vi "Redetection_initial detectoin.vi"(6 "Sweep #":i32, 7 "File Paramters":T2, 9 "New Smoothing Parameter":T3, 10 "Data (1 sweep)":dbl[](array[numeric]), 11 "Polarity":T1 items=["Inward", "Outward"]) -> (1 "Sweep trace":cluster{dbl[], "X":dbl[]}[](array[cluster]), 2 "Detected event":cluster{dbl[][]}, 3 "Original trace (unfiltered)":cluster{dbl[], "Data (1 sweep) ":dbl[]})   [LabVIEW 2017]
uses:
  Polarity.ctl
  <vilib>/Analysis/3filter.llb/Savitzky-Golay Filter (DBL).vi
  <vilib>/addons/Wavelet Analysis/application.llb/WA Multiscale Peak Detection (Array).vi
  <vilib>/Analysis/NI_AALBase.lvlib
  <vilib>/addons/_Advanced Signal Processing/NI_AdvSigProcWA.lvlib
  <vilib>/Analysis/NI_AALPro.lvlib
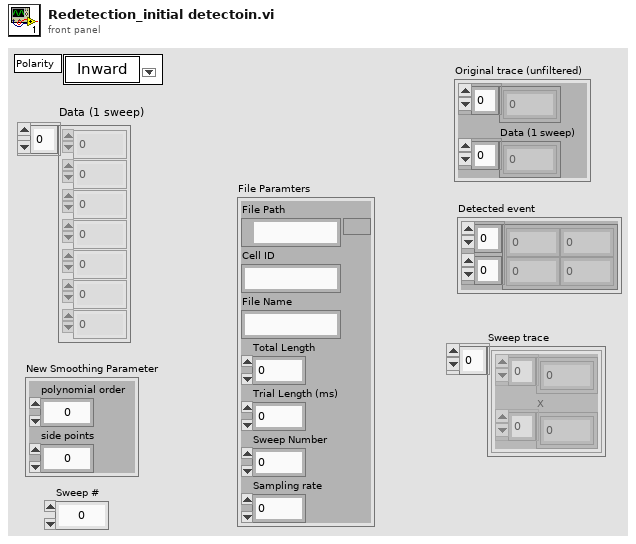
[diagram p1: front panel]
types:
  T1 = typedef "Polarity.ctl" = u16
  T2 = cluster{"File Path":path, "Cell ID":string, "File Name":string, "Total Length":i32, "Trial Length (ms)":dbl, "Sweep Number":dbl, "Sampling rate":dbl}
  T3 = cluster{"polynomial order":i32, "side points":i32}
  T4 = cluster{"detrend? (F)":bool, "threshold frequency":dbl}
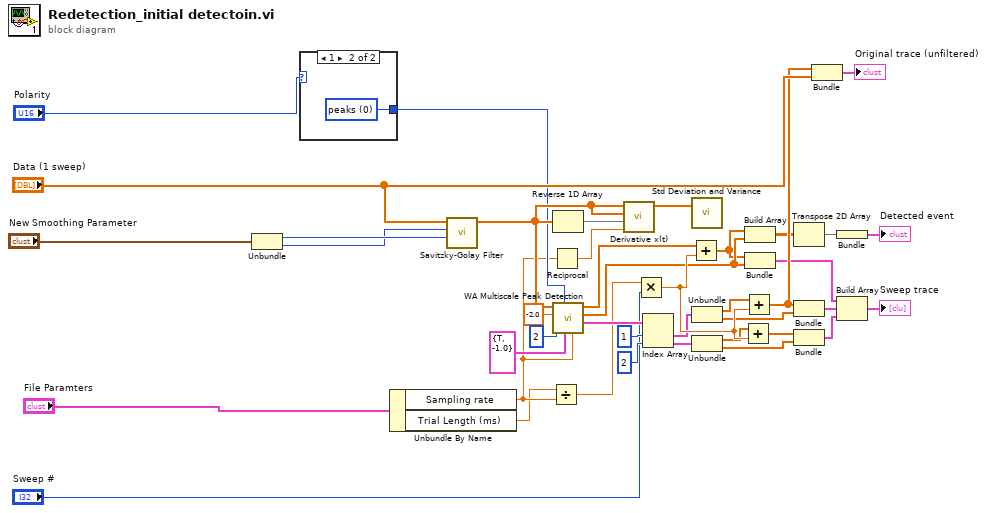
[diagram p0: block diagram]
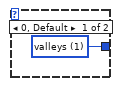
[diagram p2: hidden frame]
diagram:
  n1 = Unbundle("New Smoothing Parameter") -> ("polynomial order"=w12:i32, "side points"=w11:i32)
  n2 = case shown="1" "Polarity" {
    tunnel: [w42 w43] -> w14
    frame 0, Default {
      w42 = u16 1 items=["peaks", "valleys"] ("peaks/valleys")
    }
    frame 1 {
      w43 = u16 0 items=["peaks", "valleys"] ("peaks/valleys")
    }
  }
  n3 = Unbundle By Name("File Paramters") -> ("Sampling rate"=w9:dbl, "Trial Length (ms)"=w8:dbl)
  n4 = call-poly <vilib>:"Savitzky-Golay Filter.vi"("polynomial order"=w12, "side points"=w11, "X"="Data (1 sweep)") -> ("Filtered X"=w38:dbl[])  [unwired: 7 in, 1 out]
  n5 = Divide(x=w8, y=w9) -> (x/y=w16:dbl)
  n6 = Reciprocal(x=w9) -> (1/x=w40:dbl)
  n7 = Reverse 1D Array(array=w38) -> (reversed array=w39:dbl[])
  n8 = call-poly <vilib>:"WA Multiscale Peak Detection.vi"("sampling rate"=w9, "detrend settings"=T4 {"detrend? (F)"=TRUE, "threshold frequency"=-1.0}, "peaks/valleys"=w14, "width"=2, "threshold"=-2.0, "signal"=w38) -> ("peak plot"=w22:cluster{"Ramp Pattern":dbl[], "X":dbl[]}[], "amplitude"=w21:dbl[], "location"=w17:dbl[])  [unwired: 1 in, 2 out]
  n9 = call <vilib>:"Derivative x(t).vi"("dt"=w40, "Final Condition"=w39, "Initial Condition"=w38, "X"=w38) -> ("dX/dt"=w41:dbl[])  [unwired: 6 in, 1 out]
  n10 = Multiply(x=w16, y="Sweep #") -> (x*y=w35:dbl)
  n11 = Index Array(array=w22, index #1=1 ("인덱스"), index #2=2 ("인덱스")) -> (element #1=w24:cluster{"Ramp Pattern":dbl[], "X":dbl[]}, element #2=w28:cluster{"Ramp Pattern":dbl[], "X":dbl[]})
  n12 = Add(x=w17, y=w35) -> (x+y=w20:dbl[])
  n13 = call <vilib>:"Std Deviation and Variance.vi"("X"=w41) -> ()  [unwired: 1 in, 3 out]
  n14 = Unbundle(w24) -> ("Ramp Pattern"=w25:dbl[], "X"=w26:dbl[])
  n15 = Unbundle(w28) -> ("Ramp Pattern"=w29:dbl[], "X"=w31:dbl[])
  n16 = Add(x=w29, y=w35) -> (x+y=w30:dbl[])
  n17 = Add(x=w25, y=w35) -> (x+y=w36:dbl[])
  n18 = Build Array(w20, w21) -> (w18:dbl[][])
  n19 = Bundle(w20, "amplitude"=w21) -> (w34:cluster{dbl[], "amplitude":dbl[]})  [unwired: 1 in]
  n20 = Transpose 2D Array(2D array=w18) -> (transposed array=w19:dbl[][])
  n21 = Bundle(w36, "X"=w26) -> (w33:cluster{dbl[], "X":dbl[]})  [unwired: 1 in]
  n22 = Bundle(w30, "X"=w31) -> (w32:cluster{dbl[], "X":dbl[]})  [unwired: 1 in]
  n23 = Bundle(w36, "Data (1 sweep)"="Data (1 sweep)") -> (→"Original trace (unfiltered)":cluster{dbl[], "Data (1 sweep) ":dbl[]})  [unwired: 1 in]
  n24 = Bundle(w19) -> (→"Detected event":cluster{dbl[][]})  [unwired: 1 in]
  n25 = Build Array(w34, w33, w32) -> (→"Sweep trace":cluster{dbl[], "X":dbl[]}[])
